vi "solar_tcp Close.vi"(6 "Suppress Errors? (T)":bool=TRUE, 8 "error in (no error)":errorcluster, 10 "Shutdown? (F = Close)":bool, 11 "TCP Data in":T1={"Connected"=FALSE, "Config"={"TCPServer"=enum."SERVER", "ServerPort"=0, "IPAddress"="", "ClientPort"=0, "HdrSizeBytes"=4, "HdrLenSubtractBytes"=0, "HdrLenOffsetBits"=0, "HdrLenSizeBits"=32}, "Clients"=[], "ConnectionID"=refnum, "Debug"=[]} {"Debug"."Time" format="%<%Y-%m-%d\n%H:%M:%S%3u>T"}) -> (0 "error out":errorcluster, 3 "TCP Data out":T1 {"Debug"."Time" format="%<%Y-%m-%d\n%H:%M:%S%3u>T"})   [LabVIEW 2018]
doc: "Close or shutdown a TCP connection. Set <b>Shutdown</b> to true to close the TCP Server listener connection."
uses:
  solar_tcp_ctl Action.ctl
  solar_tcp_ctl Data.ctl
  solar_tcp_ctl Config.ctl
  solar_tcp_ctl Debug.ctl
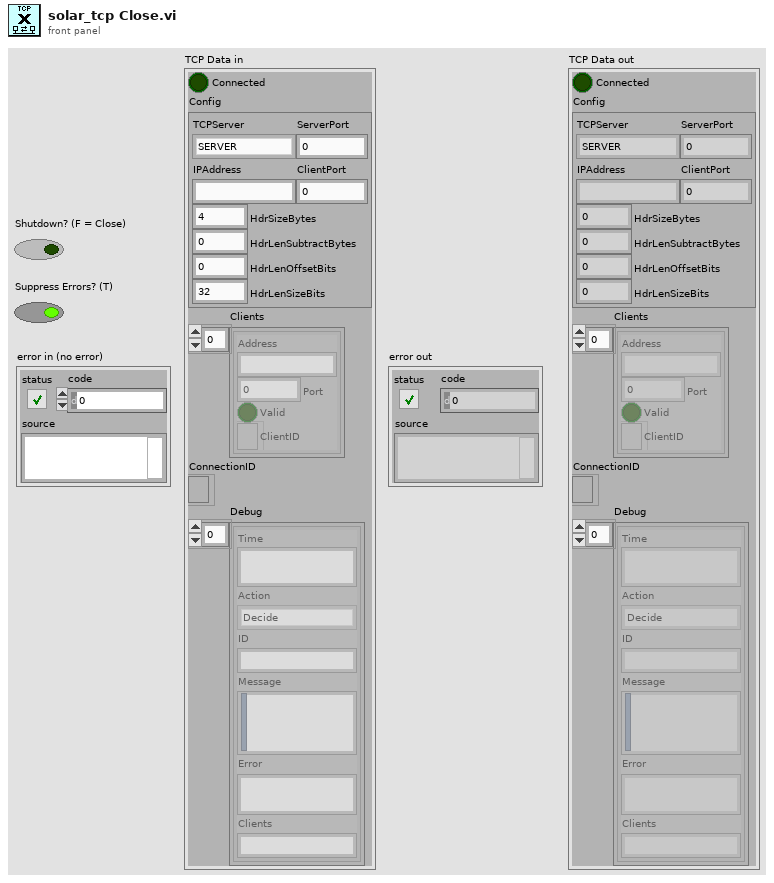
[diagram p1: front panel]
types:
  T1 = typedef "solar_tcp_ctl Data.ctl" = cluster{"Connected":bool, "Config":T2, "Clients":cluster{"Address":string, "Port":u16, "Valid":bool, "ClientID":refnum<k5>}[], "ConnectionID":refnum<k5>, "Debug":T3[]}
  T2 = typedef "solar_tcp_ctl Config.ctl" = cluster{"TCPServer":enum8{"SERVER", "CLIENT"}, "ServerPort":u16, "IPAddress":string, "ClientPort":u16, "HdrSizeBytes":i32, "HdrLenSubtractBytes":i32, "HdrLenOffsetBits":i32, "HdrLenSizeBits":i32}
  T3 = typedef "solar_tcp_ctl Debug.ctl" = cluster{"Time":timestamp, "Action":T4, "ID":string, "Message":string, "Error":string, "Clients":string}
  T4 = typedef "solar_tcp_ctl Action.ctl" = enum16{"Decide", "CreateListener", "Open", "Read", "Write", "Close", "Shutdown", "Done", "ChangePort"}
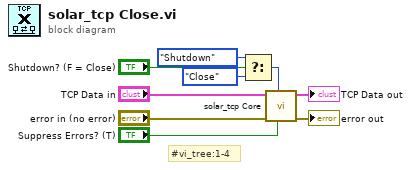
[diagram p0: block diagram]
diagram:
  # "#vi_tree:1-4"
  n1 = Select(t=solar_tcp_ctl_Action."Shutdown" ("Action"), s="Shutdown? (F = Close)", f=solar_tcp_ctl_Action."Close" ("Action")) -> (s? t:f=w2:T4)
  n2 = call "solar_tcp Core.vi"("Suppress Errors? (T)"="Suppress Errors? (T)", "Action"=w2, "error in (no error)"="error in (no error)", "TCP Data in"="TCP Data in") -> ("error out"=→"error out":errorcluster, "TCP Data out"=→"TCP Data out":T1)  [unwired: 4 in, 2 out]
